vi "OE2031&OE2041_Query PLL&Overload.vi"(0 "VISA resource name":refnum<visa-resource-name>, 5 "Connection ID in":refnum<k5>, 7 "Timeout":u32=1000, 9 "Remote Mode":u16(ring) items=["USB"=0, "RS232"=1, "Ethernet"=3], 11 "Error in (no error)":errorcluster caption="error out（no error）") -> (4 "VISA resource  out":refnum<visa-resource-name>, 6 "Connection ID out":refnum<k5>, 8 "OE2041_Query PLL&Overload":T1, 10 "Output String":string, 15 "Error out":errorcluster caption="error out")   [LabVIEW 2011]
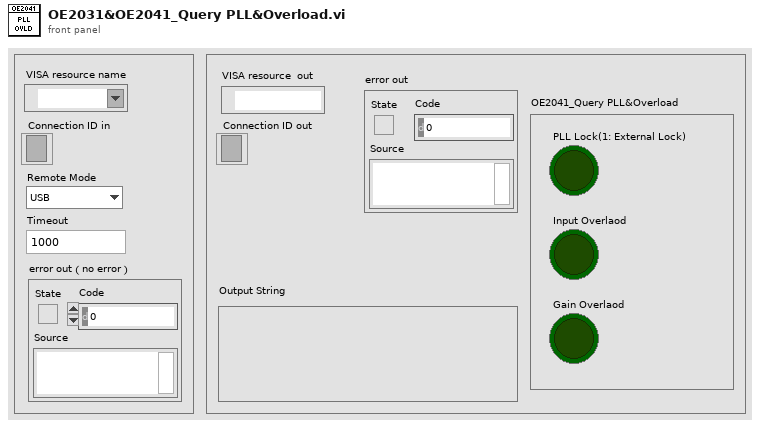
[diagram p1: front panel]
types:
  T1 = cluster{"PLL Lock(1: External Lock)":bool, "Input Overlaod":bool, "Gain Overlaod":bool}
  T2 = enum16{"ISRC", "IGND", "ICPL", "ILIN", "PHAS", "FMOD", "RSLP", "FREQ", "SWPT", "SLLM", "SULM", "SSLL", "SSLG", "STLM", "SWRM", "IRNG", "SENS", "RMOD", "OFLT", "OFSL", "SYNC", "DMOD", "HARM", "DARB", "SWVT", "SLVL", "SVLL", "SVUL", "SVSL", "SVSG", "SVTM", "SVRM", "RALL", "SNAP", "OUTP", "OAUX", "COUT", "CAUX", "COFP", "CEXP", "FPOP", "OEXP", "*IDN", "*RST", "OVLD", "INOV", "GNOV", "*PLL", "SSET", "RSET", "AGAN", "APHS", "ARSV", "ASCL", "EQCD", "EQCS", "SPED", "SRAT", "SLEN", "SSLE", "STRG", "SPRM", "STRD", "PAUS", "REST", "SPTS", "TRCA", "TEMP", "RSTU", "IHNZ", "DEQU", "SADD", "ARNG", "CSPE", "ISRCD", "IGNDD", "ICPLD", "ILIND", "PHASD", "FMODD", "RSLPD", "FREQD", "SWPTD", "SLLMD", "SULMD", "SSLLD", "SSLGD", "STLMD", "SWRMD", "SENSD", "RMODD", "OFLTD", "OFSLD", "SYNCD", "HARMD", "EQCDD", "EQCSD", "SNAPD", "OUTPD", "SWVTD", "SLVLD", "SVLLD", "SVULD", "SVSLD", "SVSGD", "SVTMD", "SVRMD", "SVDCD", "ARSVD", "AGAND", "APHSD", "ASCLD", "FPOPD", "CAUXD", "OEXPD", "SPEDD", "SRATD", "SLEND", "SSLED", "STRGD", "SPRMD", "STRDD", "PAUSD", "RESTD", "SPTSD", "TRCAD", "*IDND", "*RSTD", "INOVD", "GNOVD", "*PLLD", "SSETD", "RSETD"}
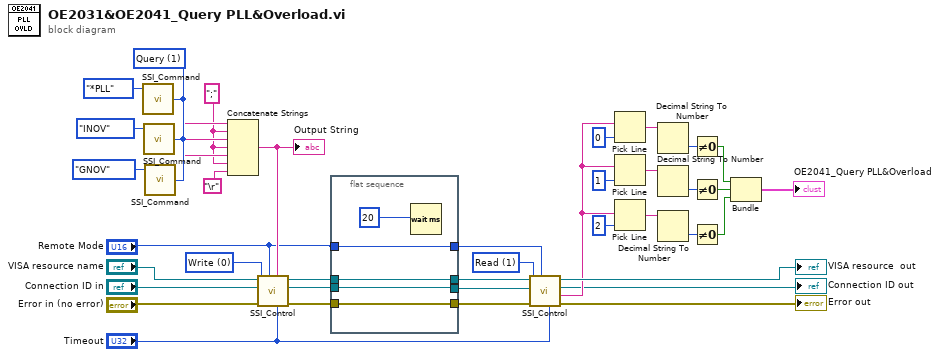
[diagram p0: block diagram]
diagram:
  w11 = ";"
  w27 = u16 1 items=["Write", "Read"] ("Control")
  w20 = u16 1 items=["Set", "Query"] ("Opera")
  w40 = u16 0 items=["Write", "Read"] ("Control")
  n1 = call "SSI_Command.vi"("Opera"=w20, "Command Type"=T2."*PLL") -> ("Output string"=w14:string)  [unwired: 2 in]
  n2 = call "SSI_Command.vi"("Opera"=w20, "Command Type"=T2."INOV") -> ("Output string"=w13:string)  [unwired: 2 in]
  n3 = call "SSI_Command.vi"("Opera"=w20, "Command Type"=T2."GNOV") -> ("Output string"=w12:string)  [unwired: 2 in]
  n4 = Concatenate Strings(w14, w11, w13, w11, w12, w11, "\r") -> (w28:string)
  "Output String" <- w28
  n5 = call "SSI_Control.vi"("Tineout"="Timeout", "Write Buffer"=w28, "Remote Mode"="Remote Mode", "Error in (no error)"="Error in (no error)", "Control"=w40, "Connection ID in"="Connection ID in", "VISA resource name"="VISA resource name") -> ("Error out"=w37:errorcluster, "Connection ID out"=w3:refnum<k5>, "VISA resource  out"=w36:refnum<visa-resource-name>)  [unwired: 1 in, 1 out]
  n6 = flat-sequence {
    tunnel: [w46] -> w35
    tunnel: w37 -> [w46]
    tunnel: [w45] -> w34
    tunnel: w36 -> [w45]
    tunnel: "Remote Mode" -> [w44]
    tunnel: [w44] -> w33
    tunnel: w3 -> [w43]
    tunnel: [w43] -> w2
    frame #0 {
      n7 = Wait (ms)(milliseconds to wait=u32 20 ("等待时间（毫秒）")) -> ()  [unwired: 1 out]
    }
  }
  n8 = call "SSI_Control.vi"("Tineout"="Timeout", "Remote Mode"=w33, "Error in (no error)"=w35, "Control"=w27, "Connection ID in"=w2, "VISA resource name"=w34) -> ("Error out"=→"Error out":errorcluster, "Read Buffer"=w17:string, "Connection ID out"=→"Connection ID out":refnum<k5>, "VISA resource  out"=→"VISA resource  out":refnum<visa-resource-name>)  [unwired: 2 in]
  n9 = Pick Line(multi-line string=w17, line index=0 ("行索引")) -> (output string=w25:string)  [unwired: 1 in]
  n10 = Pick Line(multi-line string=w17, line index=1 ("行索引")) -> (output string=w26:string)  [unwired: 1 in]
  n11 = Pick Line(multi-line string=w17, line index=2 ("行索引")) -> (output string=w19:string)  [unwired: 1 in]
  n12 = Decimal String To Number(string=w25) -> (number=w7:i32)  [unwired: 2 in, 1 out]
  n13 = Decimal String To Number(string=w26) -> (number=w8:i32)  [unwired: 2 in, 1 out]
  n14 = Decimal String To Number(string=w19) -> (number=w9:i32)  [unwired: 2 in, 1 out]
  n15 = Not Equal To 0?(x=w7) -> (x != 0?=w24:bool)
  n16 = Not Equal To 0?(x=w8) -> (x != 0?=w30:bool)
  n17 = Not Equal To 0?(x=w9) -> (x != 0?=w16:bool)
  n18 = Bundle(w24, w30, w16) -> (→"OE2041_Query PLL&Overload":cluster{bool, bool, bool})  [unwired: 1 in]
